vi "Cycle.vi"(8 "error in (no error)":errorcluster, 11 "EyeCalibration In":refnum<class "EyeCalibration.lvclass">) -> (0 "error out":errorcluster, 3 "EyeCalibration Out":refnum<class "EyeCalibration.lvclass">)   [LabVIEW 2011, in "EyeCalibration.lvclass"]
uses:
  EyeCalibration.lvclass
  Trial Based Experiment Statechart/MatlabExperiment/MatlabExperiment.lvclass
  EyeCalibration.lvclass/EyeCalibration.ctl
panel:
  in  "Fixation Radius":dbl
  out "XY Graph":cluster{"X":dbl, "Y":dbl}[](graph)
  in  "Accept Regression":bool
  out "Active Params":dbl[](array[numeric])
  out "CurrentFit":dbl[](array[numeric])
  in  "Clear Regression":bool
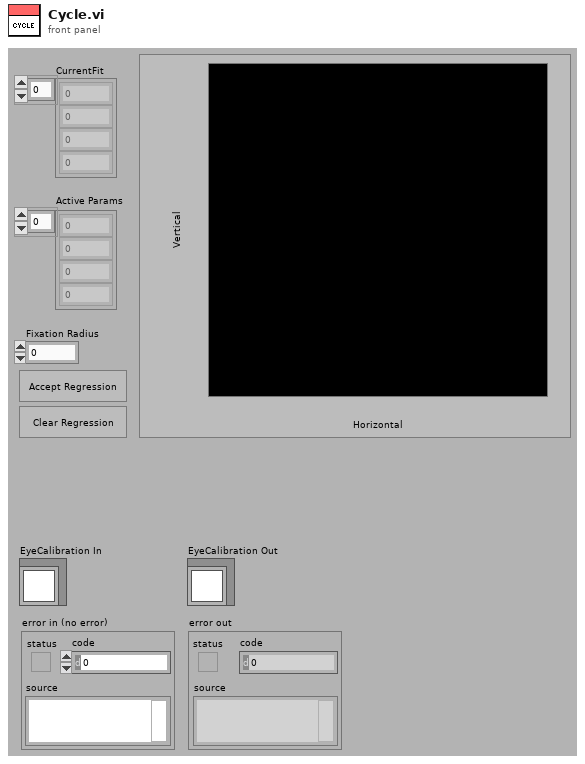
[diagram p1: front panel]
types:
  T1 = cluster{"SpotX":dbl, "SpotY":dbl, "MeasuredX":dbl, "MeasuredY":dbl}[]
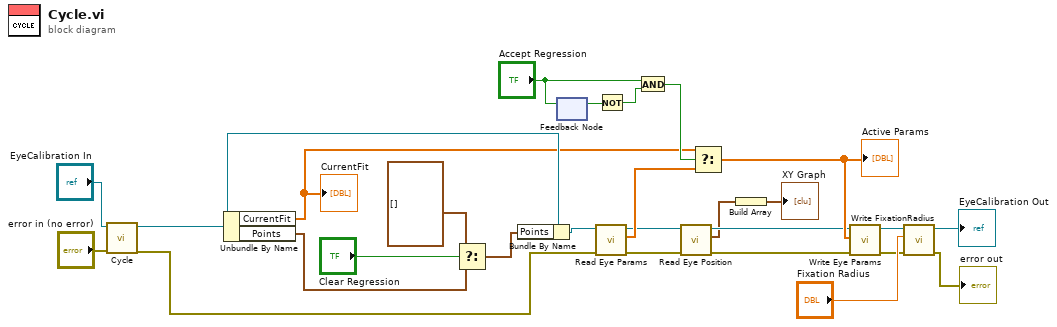
[diagram p0: block diagram]
diagram:
  n1 = call-parent "Cycle.vi"("error in (no error)"="error in (no error)", "MatlabExperiment In"="EyeCalibration In") -> ("error out"=w12:errorcluster, "MatlabExperiment Out"=w23:refnum<class "EyeCalibration.lvclass">)  [unwired: 8 in]
  n2 = Unbundle By Name(w23) -> ("CurrentFit"=w15:dbl[], "Points"=w22:T1)
  "CurrentFit" <- w15
  n3 = Select(t=T1 [], s="Clear Regression", f=w22) -> (s? t:f=w21:T1)
  n4 = Bundle By Name(cluster=w23, "Points"=w21) -> (w20:refnum<class "EyeCalibration.lvclass">)
  n5 = feedback-in #1("Accept Regression") -> ()
  n6 = feedback #1() -> (w19:bool)  [unwired: 1 in]
  n7 = call-dynamic "Read Eye Params.vi"("error in (no error)"=w12, "TrialBasedExperiment in"=w20) -> ("error out"=w9:errorcluster, "Eye Params"=w14:dbl[], "TrialBasedExperiment out"=w11:refnum<class "EyeCalibration.lvclass">)  [unwired: 7 in]
  n8 = Not(x=w19) -> (.not. x?=w18:bool)
  n9 = And(x="Accept Regression", y=w18) -> (x .and. y?=w16:bool)
  n10 = call-dynamic "Read Eye Position.vi"("error in (no error)"=w9, "TrialBasedExperiment in"=w11) -> ("error out"=w8:errorcluster, "Eye Position"=w7:cluster{"Horizontal":dbl, "Vertical":dbl}, "TrialBasedExperiment out"=w10:refnum<class "EyeCalibration.lvclass">)  [unwired: 7 in]
  n11 = Select(t=w15, s=w16, f=w14) -> (s? t:f=w13:dbl[])
  "Active Params" <- w13
  n12 = Build Array(w7) -> (→"XY Graph":cluster{"Horizontal":dbl, "Vertical":dbl}[])
  n13 = call-dynamic "Write Eye Params.vi"("error in (no error)"=w8, "Eye Params"=w13, "TrialBasedExperiment in"=w10) -> ("error out"=w2:errorcluster, "TrialBasedExperiment out"=w5:refnum<class "EyeCalibration.lvclass">)  [unwired: 7 in]
  n14 = call-dynamic "Write FixationRadius.vi"("error in (no error)"=w2, "FixationRadius"="Fixation Radius", "MatlabExperiment in"=w5) -> ("error out"=→"error out":errorcluster, "MatlabExperiment out"=→"EyeCalibration Out":refnum<class "EyeCalibration.lvclass">)  [unwired: 7 in]
